vi "Reports.Result String to State.vi"(7 "State String":string) -> (3 "Result State":T1 items=["LOG", "PASS", "FAIL", "ERROR"])   [LabVIEW 2024]
uses:
  Results/Result.Measurement and Attribute Item Status.ctl
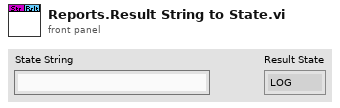
[diagram p1: front panel]
types:
  T1 = typedef "Result.Measurement and Attribute Item Status.ctl" = i32
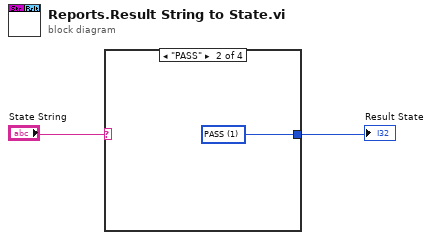
[diagram p0: block diagram]
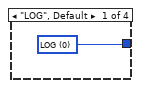
[diagram p2: hidden frame]
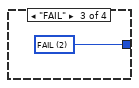
[diagram p3: hidden frame]
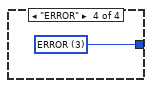
[diagram p4: hidden frame]
diagram:
  n1 = case shown="\"PASS\"" "State String" {
    tunnel: [w3 w4 w5 w6] -> w1
    frame "LOG", Default {
      w3 = T1 0 items=["LOG", "PASS", "FAIL", "ERROR"] ("Result State")
    }
    frame "PASS" {
      w4 = T1 1 items=["LOG", "PASS", "FAIL", "ERROR"] ("Result State")
    }
    frame "FAIL" {
      w5 = T1 2 items=["LOG", "PASS", "FAIL", "ERROR"] ("Result State")
    }
    frame "ERROR" {
      w6 = T1 3 items=["LOG", "PASS", "FAIL", "ERROR"] ("Result State")
    }
  }
  "Result State" <- w1
